vi "Main.vi"() -> ()   [LabVIEW 2018]
doc: "This Continuous Measurement sample project is based on the Queued Message Handler template.\n\nThe Event Handling Loop generates messages based on user interface actions.\n\nThe Message Handling Loop processes messages generated by the Event Handling Loop, or by other messages. There are also Acquisition and Logging message handling loop subVIs, and a chart updating loop."
uses:
  <vilib>/Utility/error.llb/Error Cluster From Error Code.vi
  Acquisition/Acquisition.lvlib
  support/User Event - Stop/User Event - Stop.lvlib
  support/Message Queue/Message Queue.lvlib
  support/Message Queue/Enqueue Message (Single).vi
  controls/UI State.ctl
  <vilib>/ErrorRing/Error Ring.xnode
  GlobalVariable/GlobalLongueurOnde.vi
  controls/UI Data.ctl
  GlobalVariable/GlobalSet0.vi
  GlobalVariable/GlobalDefaultFolderPath.vi
panel:
  out "Pos Y":dbl
  out "Pos X":dbl
  out "?":dbl[][](graph)
  in  "Mise à 0":bool
  in  "Longueur d'onde du laser":dbl
  in  "Exit":bool
  out "Data":waveform(dbl)[](graph)
  out "Array":variant[](array[variant])
  out "Status":string
  out "Puissance Instantannée":dbl
  in  "Start":bool
  in  "Stop":bool
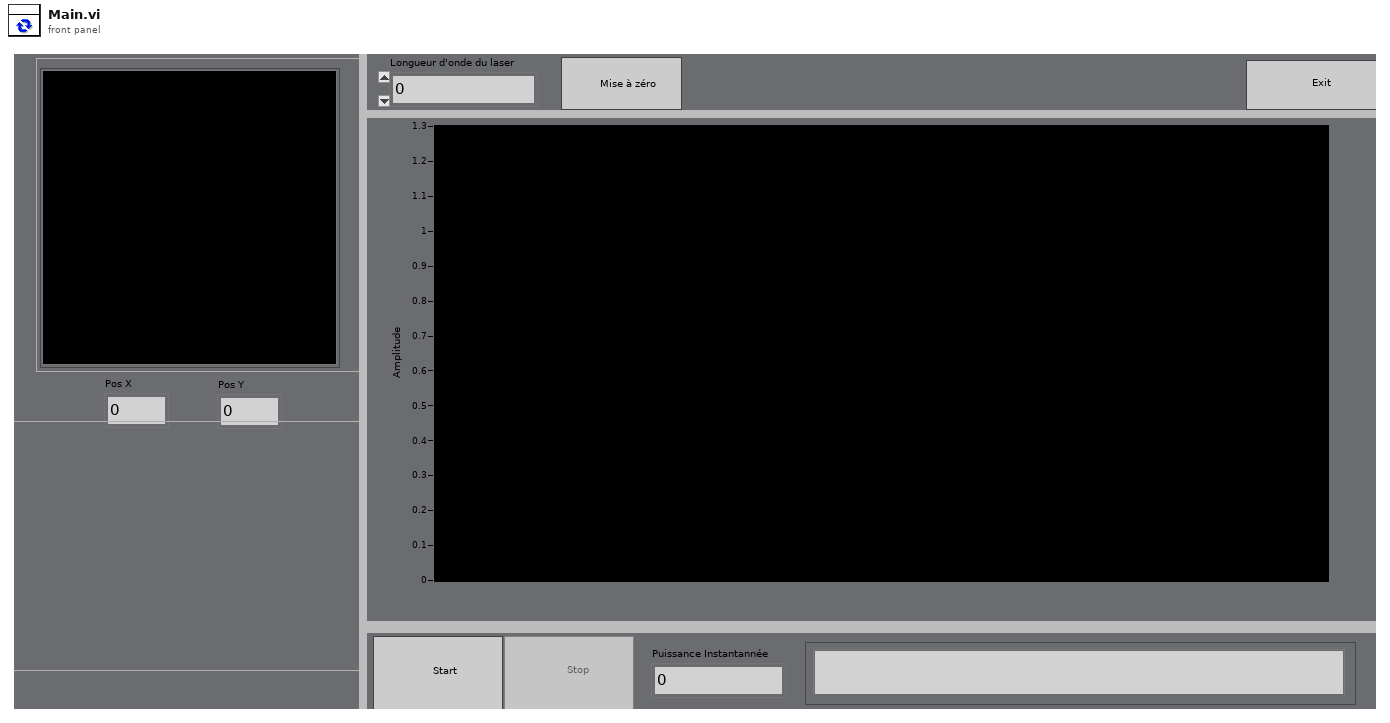
[diagram p1: front panel]
types:
  T1 = typedef "UI State.ctl" = enum16{"Idle", "Acquiring and Logging", "Waiting for Exit", "Waiting for Exit (Acq Stopped)", "Waiting for Exit (Log Stopped)", "Waiting for Stop", "Waiting for Stop (Acq Stopped)", "Waiting for Stop (Log Stopped)"}
  T2 = typedef "UI Data.ctl" = cluster{"Start Ref":refnum<vi>, "Stop Ref":refnum<vi>, "Settings Ref":refnum<vi>, "Exit Ref":refnum<vi>, "Status Ref":refnum<vi>, "Data Ref":refnum<vi>, "Longueur d'onde du laser":refnum<vi>, "Set 0 Ref":refnum<vi>}
  T3 = cluster{"UI":refnum<queue>, "Acquisition":refnum<queue>}
  T4 = enum16{"open", "replace", "create", "open or create", "replace or create", "replace or create with confirmation"}
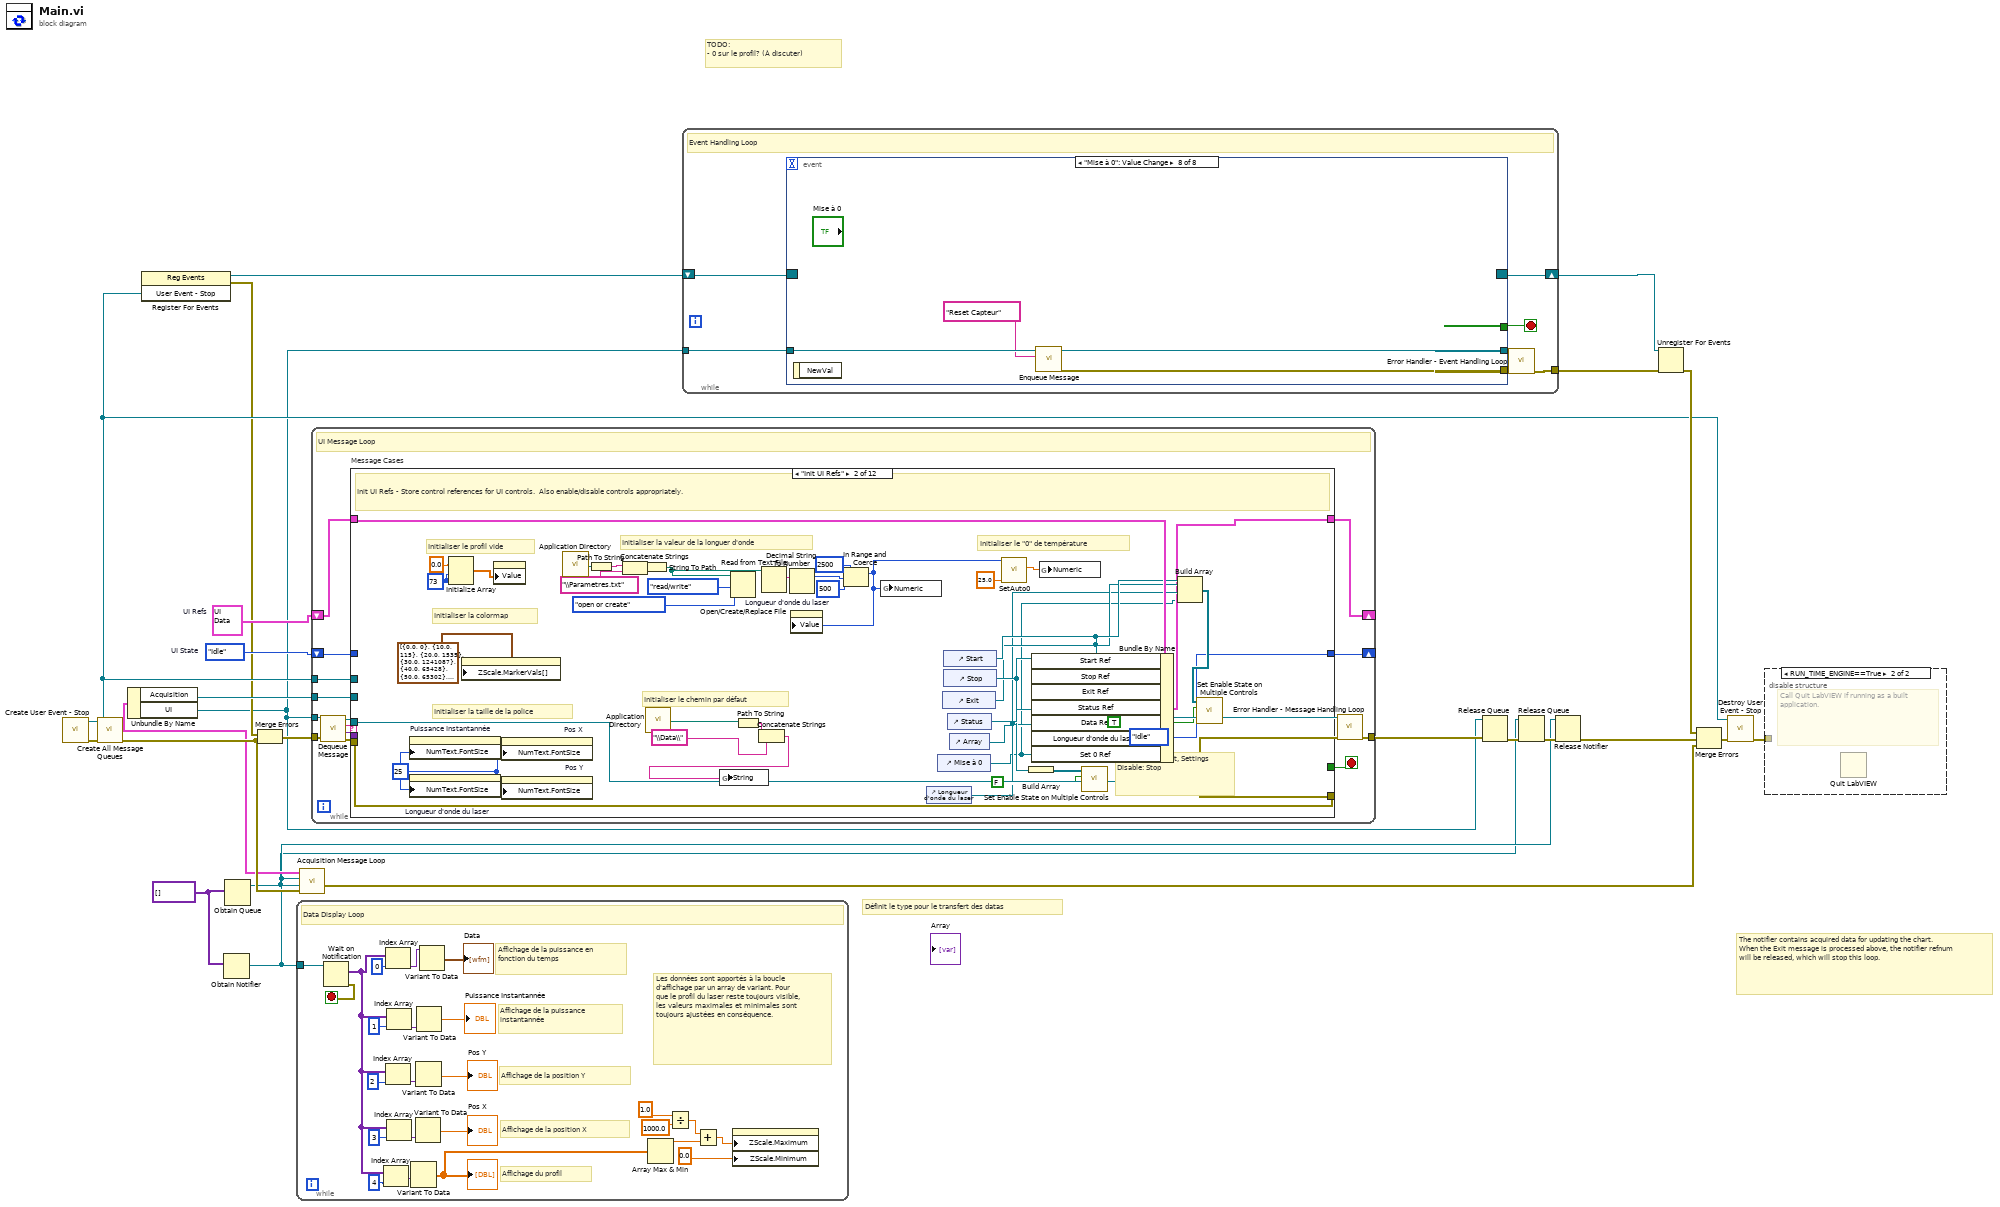
[diagram p0: block diagram]
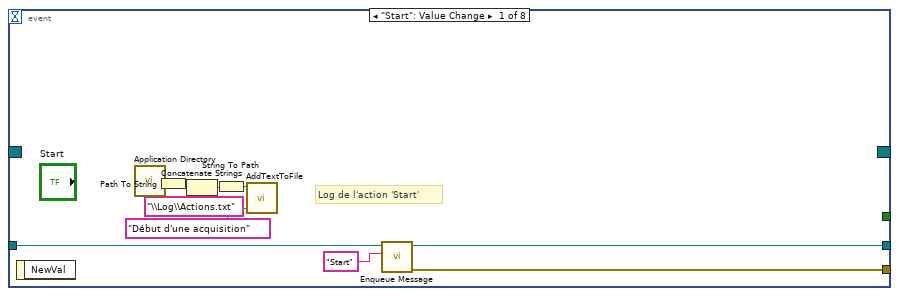
[diagram p3: hidden frame]
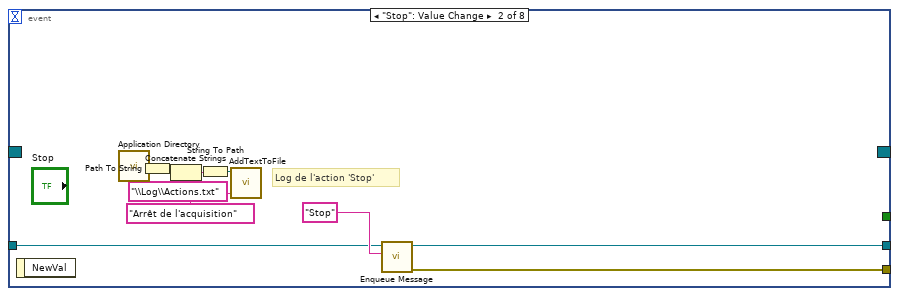
[diagram p4: hidden frame]
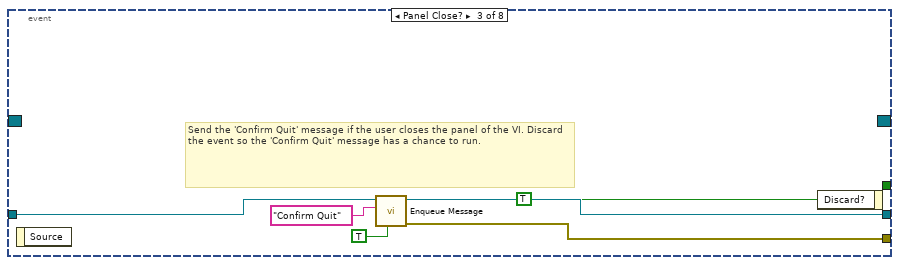
[diagram p5: hidden frame]
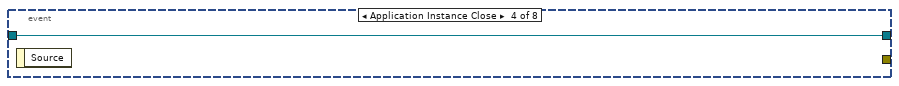
[diagram p6: hidden frame]
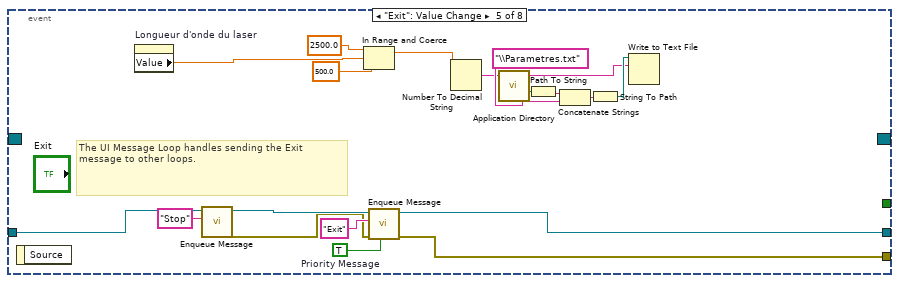
[diagram p7: hidden frame]
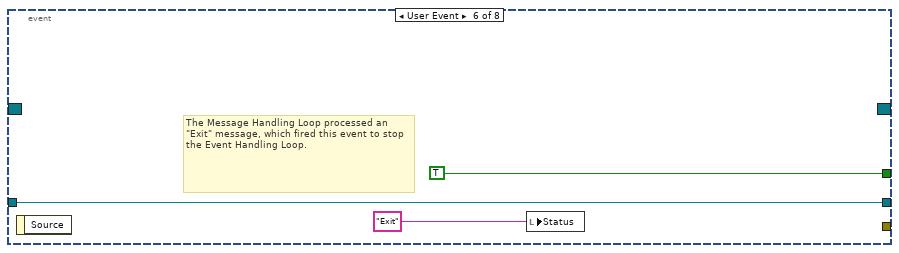
[diagram p8: hidden frame]
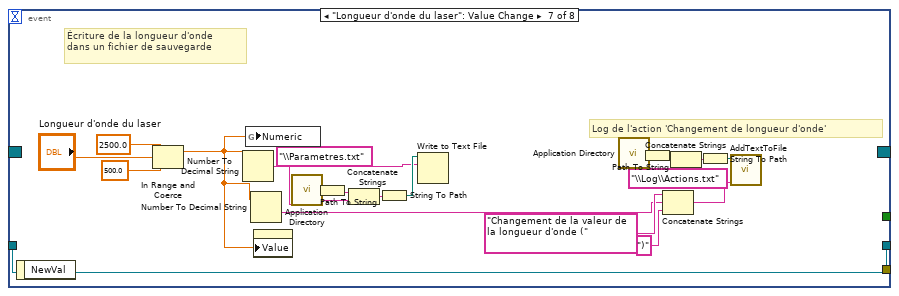
[diagram p9: hidden frame]
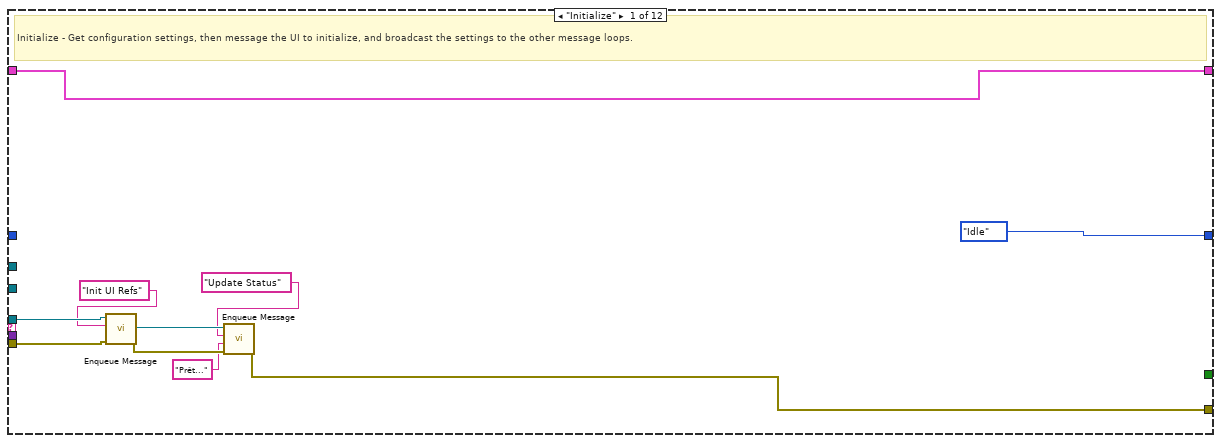
[diagram p10: hidden frame]
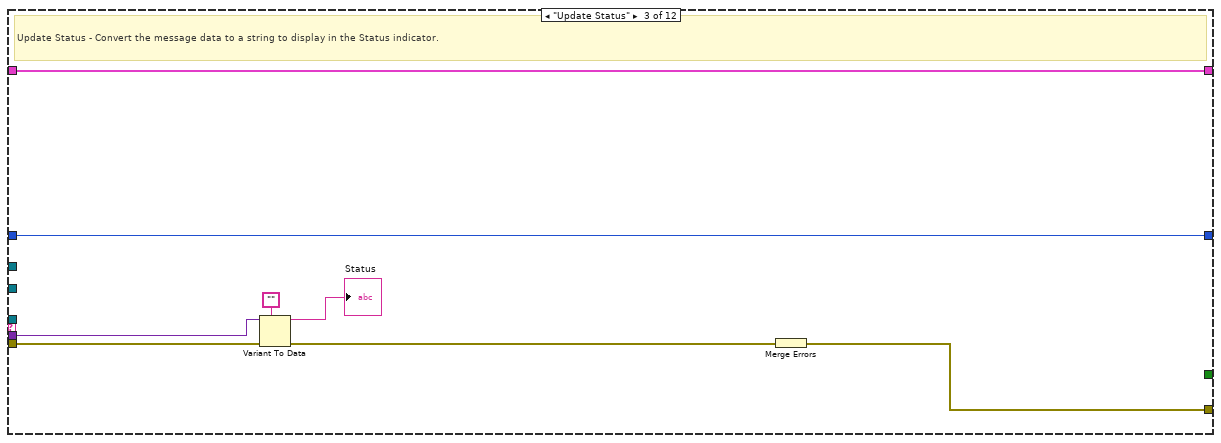
[diagram p11: hidden frame]
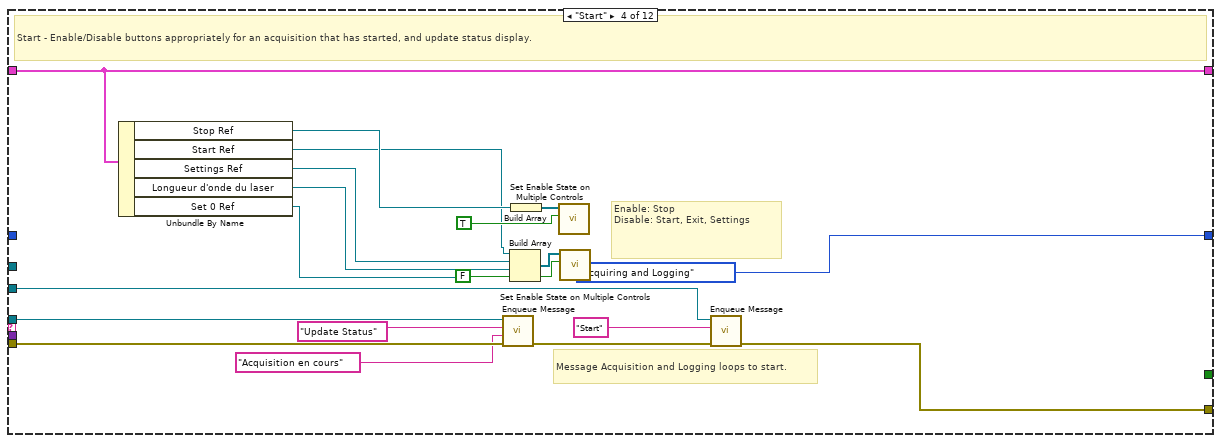
[diagram p12: hidden frame]
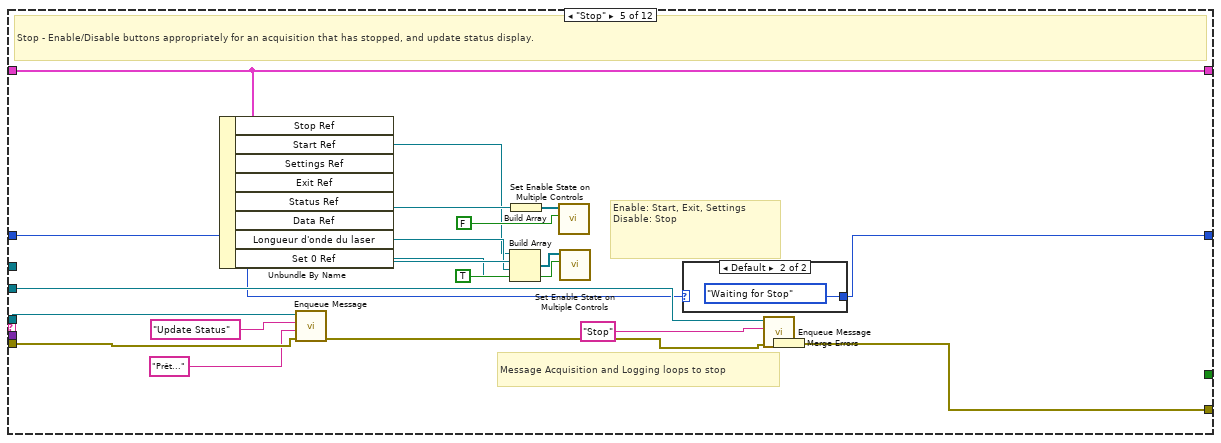
[diagram p13: hidden frame]
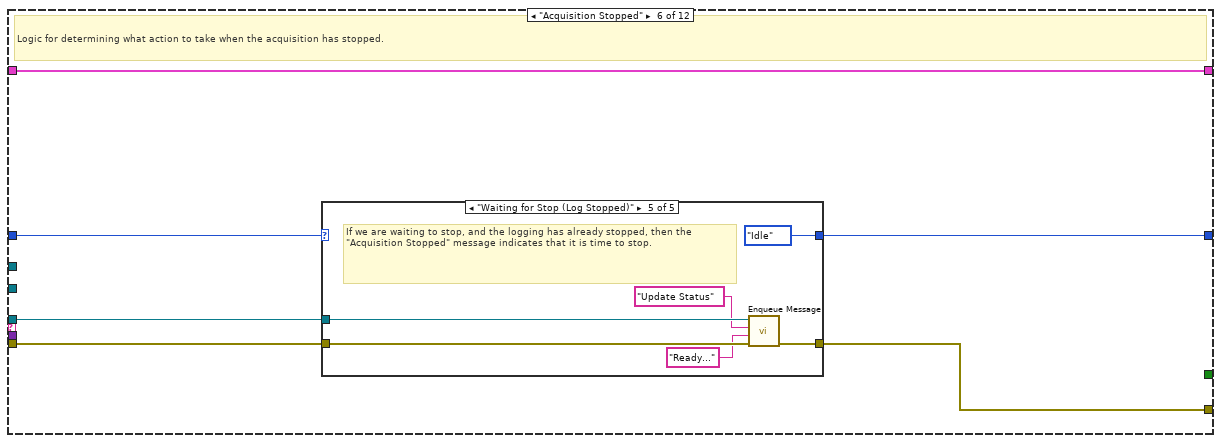
[diagram p15: hidden frame]
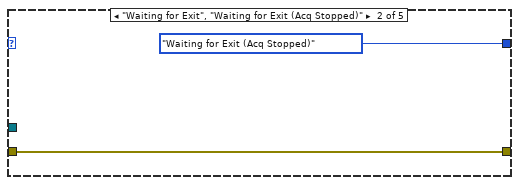
[diagram p17: hidden frame]
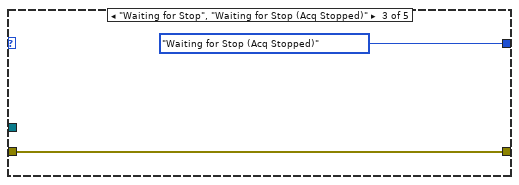
[diagram p18: hidden frame]
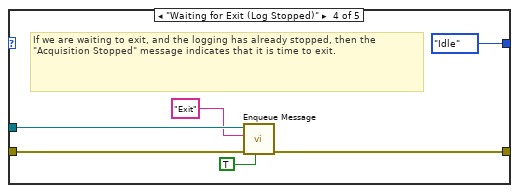
[diagram p19: hidden frame]
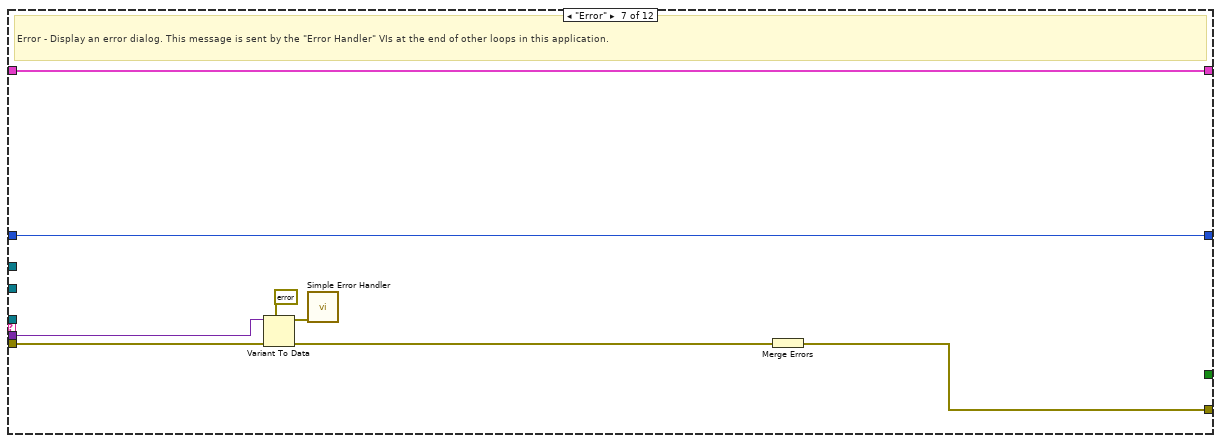
[diagram p20: hidden frame]
diagram:
  w3 = variant[] [] ("appended array")
  w16 = UI_State."Idle"  # UI State
  w18 = T2 {"Start Ref"=refnum, "Stop Ref"=refnum, "Settings Ref"=refnum, "Exit Ref"=refnum, "Status Ref"=refnum, "Data Ref"=refnum, "Longueur d'onde du laser"=refnum, "Set 0 Ref"=refnum}  # UI Refs
  # "TODO: \n- 0 sur le profil? (À discuter)"
  # "Définit le type pour le transfert des datas"
  # "The notifier contains acquired data for updating the chart. When the Exit message is processed above, the notifier refnum will be released, which will stop this loop."
  n1 = call "Create User Event - Stop.vi"() -> ("error out"=w21:errorcluster, "User Event - Stop"=w9:refnum<user-event>)  [unwired: 10 in]
  n2 = call "Create All Message Queues.vi"("error in (no error)"=w21) -> ("error out"=w20:errorcluster, "Message Queues out"=w4:T3)  [unwired: 9 in]
  n3 = Unbundle By Name(w4) -> ("Acquisition"=w17:refnum<queue>, "UI"=w6:refnum<queue>)
  n4 = register-events(w9) -> (reference out=w10:refnum<event-registration>, error out=w7:errorcluster)  [unwired: 2 in]
  n5 = Obtain Notifier(notification data type=w3) -> (notifier out=w2:refnum<notifier>)  [unwired: 3 in, 2 out]
  n6 = Obtain Queue(element data type=w3) -> (queue out=w1:refnum<queue>)  [unwired: 4 in, 2 out]
  n7 = Merge Errors(w7, w20) -> (w8:errorcluster)
  n8 = while "Data Display Loop" {
    tunnel: w2 -> [w48]
    stop <- w47 stop-if-true
    # "Les données sont apportés à la boucle d'affichage par un array de variant. Pour que le profil du laser reste toujours visible, les valeurs maximales et minimales sont toujours ajustées en conséquence."
    # "Affichage de la puissance en fonction du temps"
    # "Affichage de la position X"
    # "Affichage de la position Y"
    # "Affichage de la puissance\ninstantannée"
    # "Affichage du profil"
    # "Data Display Loop"
    n9 = Wait on Notification(notifier=w48) -> (notification=w35:variant[], error out=w47:errorcluster)  [unwired: 3 in, 2 out]
    n10 = Index Array(array=w35, index=4) -> (element=w33:variant)
    n11 = Index Array(array=w35, index=0) -> (element=w44:variant)
    n12 = Index Array(array=w35, index=2) -> (element=w39:variant)
    n13 = Index Array(array=w35, index=1) -> (element=w41:variant)
    n14 = Index Array(array=w35, index=3) -> (element=w36:variant)
    n15 = Variant To Data(Variant=w33) -> (data=w25:dbl[][])  [unwired: 2 in, 1 out]
    "?" <- w25
    n16 = Variant To Data(Variant=w36) -> (data=→"Pos X":dbl)  [unwired: 2 in, 1 out]
    n17 = Variant To Data(Variant=w39) -> (data=→"Pos Y":dbl)  [unwired: 2 in, 1 out]
    n18 = Variant To Data(Variant=w41) -> (data=→"Puissance Instantannée":dbl)  [unwired: 2 in, 1 out]
    n19 = Variant To Data(Variant=w44) -> (data=→"Data":waveform(dbl)[])  [unwired: 2 in, 1 out]
    n20 = Array Max & Min(array=w25) -> (max value=w31:dbl)  [unwired: 3 out]
    n21 = Divide(x=1.0, y=1000.0) -> (x/y=w30:dbl)
    n22 = Add(x=w30, y=w31) -> (x+y=w32:dbl)
    n23 = property class="IntGraph (strict)"("ZScale.Maximum"=w32, "ZScale.Minimum"=0.0 ("Z Scale.Range:Minimum")) -> ()  [unwired: 2 in, 2 out]
  }
  n24 = call "Acquisition Message Loop.vi"("error in (no error)"=w20, "queue out"=w1, "Data Notifier"=w2, "Message Queues"=w4) -> ("error out"=w22:errorcluster)  [unwired: 7 in]
  n25 = while {
    tunnel: w6 -> [w57]
    tunnel: w9 -> [w62]
    shift-right: [w55] -> _
    shift-left: w18 -> [w56]
    tunnel: w17 -> [w54]
    shift-right: [w49] -> _
    shift-left: w16 -> [w50]
    tunnel: w8 -> [w61]
    tunnel: [w53] -> w24
    stop <- w63 stop-if-true
    # "UI Message Loop"
    n26 = call "Dequeue Message.vi"("error in (no error)"=w61, "Message Queue"=w57) -> ("error out"=w60:errorcluster, "Message Data"=w58:variant, "Message"=w59:string, "dup Message Queue"=w51:refnum<queue>)  [unwired: 6 in]
    n27 = case "Message Cases" shown="\"Init UI Refs\"" w59 {
      selector: w59 -> [_ _ _ _ _ _ _ _ _ _ _ w275]
      tunnel: w51 -> [w68 _ _ w138 w144 w164 _ w197 _ _ w244 _]
      tunnel: w60 -> [w67 w111 w118 w137 w142 w165 w186 w196 _ w236 w243 _]
      tunnel: [w65 w111 w119 w127 w159 w162 w189 w195 w230 w235 w238 w274] -> w52
      tunnel: [_ _ _ _ _ _ _ _ TRUE _ _ _] -> w63
      tunnel: w58 -> [_ _ w117 _ _ _ w190 _ w225 _ _ _]
      tunnel: w62 -> [_ _ _ _ _ _ _ _ w231 _ _ _]
      tunnel: w56 -> [w69 w110 w113 w134 w158 w167 w193 w199 w229 w234 w237 w277]
      tunnel: [w69 w97 w113 w134 w158 w167 w193 w199 w229 w234 w237 w277] -> w55
      tunnel: w54 -> [_ _ _ w126 w150 _ _ _ w222 _ _ _]
      tunnel: w50 -> [_ _ w112 _ w147 w166 w188 w198 _ w233 w245 w276]
      tunnel: [UI_State."Idle" ("UI State") UI_State."Idle" ("UI State") w112 UI_State."Acquiring and Logging" ("UI State") w148 w163 w188 w194 UI_State."Idle" ("UI State") w233 w245 w276] -> w49
      frame "Initialize" {
        # "Initialize - Get configuration settings, then message the UI to initialize, and broadcast the settings to the other message loops."
        n28 = call-poly "Enqueue Message.vi"("error in (no error)"=w67, "Message"="Init UI Refs", "Message Queue"=w68) -> ("error out"=w73:errorcluster, "dup Message Queue"=w72:refnum<queue>)  [unwired: 7 in]
        n29 = call-poly "Enqueue Message.vi"("error in (no error)"=w73, "Message Data"="Prêt..." ("Ready..."), "Message"="Update Status", "Message Queue"=w72) -> ("error out"=w65:errorcluster)  [unwired: 6 in, 1 out]
      }
      frame "Init UI Refs" {
        w86 = 73 ("dimension size")
        w99 = 25
        # "Initialiser le \"0\" de température"
        # "Initialiser le profil vide"
        # "Initialiser la valeur de la longuer d'onde"
        # "Initialiser le chemin par défaut"
        # "Initialiser la colormap"
        # "Initialiser la taille de la police"
        # "Enable: Start, Exit, Settings\nDisable: Stop"
        # "Init UI Refs - Store control references for UI controls.  Also enable/disable controls appropriately."
        n30 = property on="Puissance Instantannée" class="DigNum (strict)"("NumText.FontSize"=w99) -> ()  [unwired: 2 in, 2 out]
        n31 = property on="Longueur d'onde du laser" class="DigNum (strict)"("NumText.FontSize"=w99) -> ()  [unwired: 2 in, 2 out]
        n32 = Initialize Array(0.0 ("element"), w86, w86) -> (w85:dbl[][])
        n33 = property class="IntGraph (strict)"("ZScale.MarkerVals[]"=cluster{dbl, u32}[] [{0.0, 0}, {10.0, 115}, {20.0, 1535}, {30.0, 1241087}, {40.0, 65428}, {50.0, 65302}, {60.0, 15925010}, {70.0, 16756736}, {80.0, 16739858}, {90.0, 16712704}, {100.0, 10420224}] ("Z Scale.Marker Values[]")) -> ()  [unwired: 2 in, 2 out]
        n34 = property class="IntGraph (strict)"("Value"=w85) -> ()  [unwired: 2 in, 2 out]
        n35 = property on="Pos X" class="DigNum (strict)"("NumText.FontSize"=w99) -> ()  [unwired: 2 in, 2 out]
        n36 = property on="Pos Y" class="DigNum (strict)"("NumText.FontSize"=w99) -> ()  [unwired: 2 in, 2 out]
        n37 = call <vilib>:"Application Directory.vi"() -> ("Application Directory"=w93:path)
        n38 = Path To String(path=w93) -> (string=w92:string)
        n39 = Concatenate Strings(w92, "\\Parametres.txt") -> (w91:string)
        n40 = String To Path(string=w91) -> (path=w79:path)
        n41 = call <vilib>:"Application Directory.vi"() -> ("Application Directory"=w96:path)
        n42 = Open/Create/Replace File(file path (use dialog)=w79, operation (0:open)=T4."open or create", access (0:read/write)=enum16{"read/write", "read-only", "write-only"}."read/write") -> ()  [unwired: 3 in, 3 out]
        n43 = Path To String(path=w96) -> (string=w95:string)
        n44 = Concatenate Strings(w95, "\\Data\\") -> (w83:string)
        n45 = global write "GlobalDefaultFolderPath.vi" "String"(w83) -> ()
        n46 = Read from Text File(file (use dialog)=w79) -> (text=w89:string)  [unwired: 3 in, 3 out]
        n47 = Decimal String To Number(string=w89) -> (number=w82:i32)  [unwired: 2 in, 1 out]
        n48 = In Range and Coerce(upper limit=2500, x=w82, lower limit=500) -> (coerced(x)=w74:i32)  [unwired: 1 out]
        n49 = property on="Longueur d'onde du laser" class="DigNum (strict)"("Value"=w74) -> ()  [unwired: 2 in, 2 out]
        n50 = global write "GlobalLongueurOnde.vi" "Numeric"(w74) -> ()
        n51 = control-ref of="Longueur d'onde du laser"() -> (w100:refnum<vi>)
        n52 = control-ref of="Mise à 0"() -> (w84:refnum<vi>)
        n53 = control-ref of="Exit"() -> (w102:refnum<vi>)
        n54 = control-ref of="Start"() -> (w103:refnum<vi>)
        n55 = control-ref of="Stop"() -> (w104:refnum<vi>)
        n56 = control-ref of="Status"() -> (w109:refnum<vi>)
        n57 = control-ref of="Array"() -> (w88:refnum<vi>)
        n58 = call "SetAuto0.vi"("Temp Ambiant"=25.0, "Longueur d'onde"=w74) -> ("0 à température ambiante"=w76:dbl)  [unwired: 9 in]
        n59 = Build Array(w104) -> (w106:refnum<vi>[])
        n60 = Bundle By Name(cluster=w110, "Start Ref"=w103, "Stop Ref"=w104, "Exit Ref"=w102, "Status Ref"=w109, "Data Ref"=w88, "Longueur d'onde du laser"=w100, "Set 0 Ref"=w84) -> (w97:T2)
        n61 = global write "GlobalSet0.vi" "Numeric"(w76) -> ()
        n62 = call "Set Enable State on Multiple Controls.vi"("Enable?"=FALSE, "Controls"=w106) -> ()  [unwired: 10 in]
        n63 = Build Array(w103, w102, w100, w84) -> (w107:refnum<vi>[])
        n64 = call "Set Enable State on Multiple Controls.vi"("Enable?"=TRUE, "Controls"=w107) -> ()  [unwired: 10 in]
      }
      frame "Update Status" {
        # "Update Status - Convert the message data to a string to display in the Status indicator."
        n65 = Variant To Data(error in=w118, type="", Variant=w117) -> (data=→"Status":string, error out=w115:errorcluster)
        n66 = Merge Errors(w115) -> (w119:errorcluster)
      }
      frame "Start" {
        # "Message Acquisition and Logging loops to start."
        # "Enable: Stop\nDisable: Start, Exit, Settings"
        # "Start - Enable/Disable buttons appropriately for an acquisition that has started, and update status display."
        n67 = Unbundle By Name(w134) -> ("Stop Ref"=w129:refnum<vi>, "Start Ref"=w122:refnum<vi>, "Settings Ref"=w128:refnum<vi>, "Longueur d'onde du laser"=w123:refnum<vi>, "Set 0 Ref"=w120:refnum<vi>)
        n68 = call-poly "Enqueue Message.vi"("error in (no error)"=w137, "Message Data"="Acquisition en cours" ("Acquiring and Logging..."), "Message"="Update Status", "Message Queue"=w138) -> ("error out"=w121:errorcluster)  [unwired: 6 in, 1 out]
        n69 = Build Array(w122, w128, w123, w120) -> (w132:refnum<vi>[])
        n70 = Build Array(w129) -> (w131:refnum<vi>[])
        n71 = call "Set Enable State on Multiple Controls.vi"("Enable?"=TRUE, "Controls"=w131) -> ()  [unwired: 10 in]
        n72 = call "Set Enable State on Multiple Controls.vi"("Enable?"=FALSE, "Controls"=w132) -> ()  [unwired: 10 in]
        n73 = call-poly "Enqueue Message.vi"("error in (no error)"=w121, "Message"="Start", "Message Queue"=w126) -> ("error out"=w127:errorcluster)  [unwired: 7 in, 1 out]
      }
      frame "Stop" {
        # "Message Acquisition and Logging loops to stop"
        # "Enable: Start, Exit, Settings\nDisable: Stop"
        # "Stop - Enable/Disable buttons appropriately for an acquisition that has stopped, and update status display."
        n74 = Unbundle By Name(w158) -> ("Stop Ref"=w153:refnum<vi>, "Start Ref"=w145:refnum<vi>, "Settings Ref"=w152:refnum<vi>, "Longueur d'onde du laser"=w146:refnum<vi>, "Set 0 Ref"=w139:refnum<vi>)  [unwired: 3 out]
        n75 = call-poly "Enqueue Message.vi"("error in (no error)"=w142, "Message Data"="Prêt..." ("Acquiring and Logging..."), "Message"="Update Status", "Message Queue"=w144) -> ("error out"=w140:errorcluster)  [unwired: 6 in, 1 out]
        n76 = Build Array(w145, w152, w146, w139) -> (w156:refnum<vi>[])
        n77 = Build Array(w153) -> (w155:refnum<vi>[])
        n78 = call "Set Enable State on Multiple Controls.vi"("Enable?"=FALSE, "Controls"=w155) -> ()  [unwired: 10 in]
        n79 = call "Set Enable State on Multiple Controls.vi"("Enable?"=TRUE, "Controls"=w156) -> ()  [unwired: 10 in]
        n80 = case shown="Default" w147 {
          selector: w147 -> [w160 _]
          tunnel: [w160 UI_State."Waiting for Stop" ("UI State")] -> w148
          frame "Waiting for Exit" {
          }
          frame Default {
          }
        }
        n81 = call-poly "Enqueue Message.vi"("error in (no error)"=w140, "Message"="Stop", "Message Queue"=w150) -> ("error out"=w151:errorcluster)  [unwired: 7 in, 1 out]
        n82 = Merge Errors(w151) -> (w159:errorcluster)
      }
      frame "Acquisition Stopped" {
        # "Logic for determining what action to take when the acquisition has stopped."
        n83 = case shown="\"Waiting for Stop (Log Stopped)\"" w166 {
          selector: w166 -> [w169 _ _ _ _]
          tunnel: w165 -> [w168 w171 w173 w179 w185]
          tunnel: w164 -> [_ _ _ w177 w182]
          tunnel: [w169 UI_State."Waiting for Exit (Acq Stopped)" ("UI State") UI_State."Waiting for Stop (Acq Stopped)" ("UI State") UI_State."Idle" ("UI State") UI_State."Idle" ("UI State")] -> w163
          tunnel: [w168 w171 w173 w178 w183] -> w162
          frame Default {
          }
          frame "Waiting for Exit", "Waiting for Exit (Acq Stopped)" {
          }
          frame "Waiting for Stop", "Waiting for Stop (Acq Stopped)" {
          }
          frame "Waiting for Exit (Log Stopped)" {
            # "If we are waiting to exit, and the logging has already stopped, then the \"Acquisition Stopped\" message indicates that it is time to exit."
            n84 = call-poly "Enqueue Message.vi"("Priority Message? (F)"=TRUE, "error in (no error)"=w179, "Message"="Exit", "Message Queue"=w177) -> ("error out"=w178:errorcluster)  [unwired: 6 in, 1 out]
          }
          frame "Waiting for Stop (Log Stopped)" {
            # "If we are waiting to stop, and the logging has already stopped, then the \"Acquisition Stopped\" message indicates that it is time to stop."
            n85 = call-poly "Enqueue Message.vi"("error in (no error)"=w185, "Message Data"="Ready..." ("Ready..."), "Message"="Update Status", "Message Queue"=w182) -> ("error out"=w183:errorcluster)  [unwired: 6 in, 1 out]
          }
        }
      }
      frame "Error" {
        # "Error - Display an error dialog. This message is sent by the \"Error Handler\" VIs at the end of other loops in this application."
        n86 = Variant To Data(error in=w186, type=errorcluster {"status"=FALSE, "code"=0, "source"=""} ("error constant"), Variant=w190) -> (data=w187:errorcluster, error out=w191:errorcluster)
        n87 = call <vilib>:"Simple Error Handler.vi"("error in (no error)"=w187) -> ()  [unwired: 4 in, 5 out]
        n88 = Merge Errors(w191) -> (w189:errorcluster)
      }
      frame "Confirm Quit" {
        # "Confirm Quit - Message that can confirm whether or not the user wants to exit the application."
        n89 = case shown="\"Acquiring and Logging\"" w198 {
          tunnel: w197 -> [w205 w209]
          tunnel: w196 -> [w204 w208]
          tunnel: [w203 w207] -> w195
          tunnel: [UI_State."Idle" ("UI State") w206] -> w194
          frame Default {
            # "If 'Confirm Quit' comes in while the system is idle, there is no need for a confirmation message."
            n90 = call-poly "Enqueue Message.vi"("Priority Message? (F)"=TRUE, "error in (no error)"=w204, "Message"="Exit", "Message Queue"=w205) -> ("error out"=w203:errorcluster)  [unwired: 6 in, 1 out]
          }
          frame "Acquiring and Logging" {
            n91 = Two Button Dialog(message="Are you sure you want to quit while the acquisition is running?" ("Confirm Quit Message"), 1:"No" ("No"), 2:"Yes" ("Yes")) -> (T button?=w210:bool)
            n92 = case shown="True" w210 {
              tunnel: w209 -> [_ w219]
              tunnel: w208 -> [w215 w220]
              tunnel: [w215 w218] -> w207
              tunnel: [UI_State."Acquiring and Logging" ("UI State") UI_State."Waiting for Exit" ("UI State")] -> w206
              frame False {
                # "User did not want to quit."
              }
              frame True {
                n93 = call-poly "Enqueue Message.vi"("error in (no error)"=w220, "Message"="Stop", "Message Queue"=w219) -> ("error out"=w218:errorcluster)  [unwired: 7 in, 1 out]
              }
            }
          }
        }
      }
      frame "Exit" {
        # "Popup an error dialog if 'Exit' was called as a result of an error."
        # "Stop the VI"
        # "Exit - Send Exit messages to the Acquisition and Logging loops, and fire the user event to stop the Event Handling Loop."
        n94 = Variant To Data(type=errorcluster {"status"=FALSE, "code"=0, "source"=""} ("error constant"), Variant=w225) -> (data=w224:errorcluster)  [unwired: 1 in, 1 out]
        n95 = call <vilib>:"Simple Error Handler.vi"("error in (no error)"=w224) -> ()  [unwired: 4 in, 5 out]
        n96 = call-poly "Enqueue Message.vi"("Priority Message? (F)"=FALSE, "Message"="Exit", "Message Queue"=w222) -> ("error out"=w221:errorcluster)  [unwired: 7 in, 1 out]
        n97 = call "Fire User Event - Stop.vi"("error in (no error)"=w221, "User Event - Stop"=w231) -> ("error out"=w230:errorcluster)  [unwired: 9 in]
      }
      frame "---Copy This Frame---" {
        # "Duplicate this frame when creating new messages.  Change this comment in the duplicated frame to describe this message."
        n98 = Merge Errors(w236) -> (w235:errorcluster)
      }
      frame "Reset Capteur" {
        # "Duplicate this frame when creating new messages.  Change this comment in the duplicated frame to describe this message."
        n99 = flat-sequence {
          tunnel: w244 -> [w258]
          tunnel: w243 -> [w257]
          tunnel: [w254] -> w242
          tunnel: [w253] -> w239
          tunnel: w237 -> [w252]
          tunnel: w242 -> [w260]
          tunnel: [w260] -> w241
          tunnel: [w259] -> w240
          tunnel: w239 -> [w259]
          tunnel: w241 -> [w273]
          tunnel: w240 -> [w272]
          tunnel: [w269] -> w238
          tunnel: w237 -> [w268]
          frame #0 {
            n100 = Unbundle By Name(w252) -> ("Stop Ref"=w251:refnum<vi>, "Start Ref"=w250:refnum<vi>, "Longueur d'onde du laser"=w249:refnum<vi>, "Set 0 Ref"=w248:refnum<vi>)
            n101 = call-poly "Enqueue Message.vi"("error in (no error)"=w257, "Message Data"="Mise à 0 en cours" ("Message"), "Message"="Update Status", "Message Queue"=w258) -> ("error out"=w253:errorcluster, "dup Message Queue"=w254:refnum<queue>)  [unwired: 6 in]
            n102 = Build Array(w251, w250, w249, w248) -> (w247:refnum<vi>[])
            n103 = call "Set Enable State on Multiple Controls.vi"("Enable?"=FALSE, "Controls"=w247) -> ()  [unwired: 10 in]
          }
          frame #1 {
            n104 = global read "GlobalLongueurOnde.vi" "Numeric"() -> (w262:dbl)
            n105 = call "SetTo0.vi"("Longueur d'onde"=w262) -> ("Température 0"=w261:dbl)  [unwired: 10 in]
            n106 = global write "GlobalSet0.vi" "Numeric"(w261) -> ()
          }
          frame #2 {
            n107 = Unbundle By Name(w268) -> ("Start Ref"=w267:refnum<vi>, "Longueur d'onde du laser"=w266:refnum<vi>, "Set 0 Ref"=w265:refnum<vi>)
            n108 = call-poly "Enqueue Message.vi"("error in (no error)"=w272, "Message Data"="Prêt..." ("Message"), "Message"="Update Status", "Message Queue"=w273) -> ("error out"=w269:errorcluster)  [unwired: 6 in, 1 out]
            n109 = Build Array(w267, w266, w265) -> (w264:refnum<vi>[])
            n110 = call "Set Enable State on Multiple Controls.vi"("Enable?"=TRUE, "Controls"=w264) -> ()  [unwired: 10 in]
          }
        }
      }
      frame Default {
        # "'Default' case only runs if there is a message that isn't defined in any of the other cases.  Output a programming error."
        n111 = xnode "Error Ring"("parameter 0"=w275) -> ("error out"=w274:errorcluster)
      }
    }
    n112 = call "Error Handler - Message Handling Loop.vi"("error in (no error)"=w52, "Message Queue"=w51) -> ("dup error in"=w53:errorcluster)  [unwired: 8 in, 1 out]
  }
  n113 = while {
    tunnel: w6 -> [w290]
    tunnel: [w287] -> w23
    shift-right: [w289] -> w5
    shift-left: w10 -> [w291]
    stop <- w288 stop-if-true
    # "Event Handling Loop"
    n114 = event shown="[7] \"Mise à 0\": Value Change" {
      selector: w291 -> [_ _ _ _ _ _ _ _]
      dyn-events: [_ _ _ _ _ _ _ _] -> w289
      timeout: _ -> [_ _ _ _ _ _ _ _]
      tunnel: [_ _ _ _ _ TRUE ("Discard?") _ _] -> w288
      tunnel: w290 -> [w301 w310 w315 w318 w332 w337 w359 w363]
      tunnel: [w299 w309 w313 _ w336 _ _ w361] -> w286
      tunnel: [w298 w308 w314 w318 w333 w337 w359 w362] -> w285
      event "Start": Value Change {
        # "Log de l'action 'Start'"
        n115 = event-data() -> ()  [unwired: 1 in, 1 out]
        n116 = call <vilib>:"Application Directory.vi"() -> ("Application Directory"=w295:path)
        n117 = Path To String(path=w295) -> (string=w296:string)
        n118 = Concatenate Strings(w296, "\\Log\\Actions.txt") -> (w297:string)
        n119 = String To Path(string=w297) -> (path=w293:path)
        n120 = call "AddTextToFile.vi"("Ajouter du texte"="Début d'une acquisition", "Fichier"=w293) -> ()  [unwired: 10 in]
        n121 = call-poly "Enqueue Message.vi"("Message"="Start", "Message Queue"=w301) -> ("error out"=w299:errorcluster, "dup Message Queue"=w298:refnum<queue>)  [unwired: 8 in]
      }
      event "Stop": Value Change {
        # "Log de l'action 'Stop'"
        n122 = event-data() -> ()  [unwired: 1 in, 1 out]
        n123 = call <vilib>:"Application Directory.vi"() -> ("Application Directory"=w305:path)
        n124 = Path To String(path=w305) -> (string=w306:string)
        n125 = Concatenate Strings(w306, "\\Log\\Actions.txt") -> (w307:string)
        n126 = String To Path(string=w307) -> (path=w303:path)
        n127 = call "AddTextToFile.vi"("Ajouter du texte"="Arrêt de l'acquisition", "Fichier"=w303) -> ()  [unwired: 10 in]
        n128 = call-poly "Enqueue Message.vi"("Message"="Stop", "Message Queue"=w310) -> ("error out"=w309:errorcluster, "dup Message Queue"=w308:refnum<queue>)  [unwired: 8 in]
      }
      event Panel Close? {
        # "Send the 'Confirm Quit' message if the user closes the panel of the VI. Discard the event so the 'Confirm Quit' message has a chance to run."
        n129 = event-data() -> ()  [unwired: 1 in, 1 out]
        n130 = call-poly "Enqueue Message.vi"("Priority Message? (F)"=TRUE, "Message"="Confirm Quit", "Message Queue"=w315) -> ("error out"=w313:errorcluster, "dup Message Queue"=w314:refnum<queue>)  [unwired: 7 in]
        n131 = event-data("Discard?"=TRUE) -> ()  [unwired: 1 in, 1 out]
      }
      event Application Instance Close {
        n132 = event-data() -> ()  [unwired: 1 in, 1 out]
      }
      event "Exit": Value Change {
        w334 = TRUE  # Priority Message
        # "The UI Message Loop handles sending the Exit message to other loops."
        n133 = event-data() -> ()  [unwired: 1 in, 1 out]
        n134 = property on="Longueur d'onde du laser" class="DigNum (strict)"() -> ("Value"=w319:dbl)  [unwired: 2 in, 2 out]
        n135 = call-poly "Enqueue Message.vi"("Message"="Stop", "Message Queue"=w332) -> ("error out"=w330:errorcluster, "dup Message Queue"=w331:refnum<queue>)  [unwired: 8 in]
        n136 = In Range and Coerce(upper limit=2500.0, x=w319, lower limit=500.0) -> (coerced(x)=w321:dbl)  [unwired: 1 out]
        n137 = call-poly "Enqueue Message.vi"("Priority Message? (F)"=w334, "error in (no error)"=w330, "Message"="Exit", "Message Queue"=w331) -> ("error out"=w336:errorcluster, "dup Message Queue"=w333:refnum<queue>)  [unwired: 6 in]
        n138 = Number To Decimal String(number=w321) -> (decimal integer string=w323:string)  [unwired: 1 in]
        n139 = call <vilib>:"Application Directory.vi"() -> ("Application Directory"=w328:path)
        n140 = Path To String(path=w328) -> (string=w327:string)
        n141 = Concatenate Strings(w327, "\\Parametres.txt") -> (w325:string)
        n142 = String To Path(string=w325) -> (path=w324:path)
        n143 = Write to Text File(file (use dialog)=w324, text=w323) -> ()  [unwired: 2 in, 3 out]
      }
      event User Event {
        # "The Message Handling Loop processed an \"Exit\" message, which fired this event to stop the Event Handling Loop."
        n144 = event-data() -> ()  [unwired: 1 in, 1 out]
        n145 = local write "Status"("Exit" ("Exit String")) -> ()
      }
      event "Longueur d'onde du laser": Value Change {
        # "Log de l'action 'Changement de longueur d'onde'"
        # "Écriture de la longueur d'onde\ndans un fichier de sauvegarde"
        n146 = event-data() -> ()  [unwired: 1 in, 1 out]
        n147 = In Range and Coerce(upper limit=2500.0, x="Longueur d'onde du laser", lower limit=500.0) -> (coerced(x)=w340:dbl)  [unwired: 1 out]
        n148 = Number To Decimal String(number=w340) -> (decimal integer string=w353:string)  [unwired: 1 in]
        n149 = global write "GlobalLongueurOnde.vi" "Numeric"(w340) -> ()
        n150 = Number To Decimal String(number=w340) -> (decimal integer string=w346:string)  [unwired: 1 in]
        n151 = property on="Longueur d'onde du laser" class="DigNum (strict)"("Value"=w340) -> ()  [unwired: 2 in, 2 out]
        n152 = call <vilib>:"Application Directory.vi"() -> ("Application Directory"=w358:path)
        n153 = Path To String(path=w358) -> (string=w357:string)
        n154 = Concatenate Strings(w357, "\\Parametres.txt") -> (w355:string)
        n155 = String To Path(string=w355) -> (path=w354:path)
        n156 = Write to Text File(file (use dialog)=w354, text=w353) -> ()  [unwired: 2 in, 3 out]
        n157 = call <vilib>:"Application Directory.vi"() -> ("Application Directory"=w350:path)
        n158 = Path To String(path=w350) -> (string=w351:string)
        n159 = Concatenate Strings("Changement de la valeur de la longueur d'onde (" ("Ajouter du texte"), w346, ")" ("string")) -> (w344:string)
        n160 = Concatenate Strings(w351, "\\Log\\Actions.txt") -> (w352:string)
        n161 = String To Path(string=w352) -> (path=w348:path)
        n162 = call "AddTextToFile.vi"("Ajouter du texte"=w344, "Fichier"=w348) -> ()  [unwired: 10 in]
      }
      event "Mise à 0": Value Change {
        n163 = event-data() -> ()  [unwired: 1 in, 1 out]
        n164 = call-poly "Enqueue Message.vi"("Message"="Reset Capteur", "Message Queue"=w363) -> ("error out"=w361:errorcluster, "dup Message Queue"=w362:refnum<queue>)  [unwired: 8 in]
      }
    }
    n165 = call "Error Handler - Event Handling Loop.vi"("error in (no error)"=w286, "Message Queue"=w285) -> ("dup error in"=w287:errorcluster)  [unwired: 8 in, 1 out]
  }
  n166 = Release Queue(queue=w6, error in (no error)=w24) -> (error out=w13:errorcluster)  [unwired: 1 in, 2 out]
  n167 = Release Queue(queue=w1, error in (no error)=w13) -> (error out=w12:errorcluster)  [unwired: 1 in, 2 out]
  n168 = Release Notifier(notifier=w2, error in (no error)=w12) -> (error out=w11:errorcluster)  [unwired: 1 in, 2 out]
  n169 = Unregister For Events(event registration refnum=w5, error in=w23) -> (error out=w19:errorcluster)
  n170 = Merge Errors(w19, w11, w22) -> (w15:errorcluster)
  n171 = call "Destroy User Event - Stop.vi"("error in (no error)"=w15, "User Event - Stop"=w9) -> ("error out"=w14:errorcluster)  [unwired: 9 in]
  n172 = disable-structure shown="RUN_TIME_ENGINE==True" {
    disable-tunnel: w14 -> [_ _]
    frame condition #0 (active) {
    }
    frame condition #1 {
      # "Call Quit LabVIEW if running as a built application."
      n173 = Quit LabVIEW() -> ()  [unwired: 1 in]
    }
  }
